vi "QuantumX_EnableBlinking.vi"(8 "Error in":errorcluster, 9 "BlinkColor":i32(ring)=2 items=["Green"=1, "Orange"=2, "Red"=3], 10 "Signal":refnum<k24>, 11 "DevicesAndSignals":T1) -> (0 "Error out":errorcluster, 3 "DevicesAndSignals":T1)   [LabVIEW 2016]
doc: "Enables blinking at the connector to which the given signal belongs.\n\nSignal: Signal, whose connector should start blinking in the given color.\nBlinkColor: Blinking color of the LED."
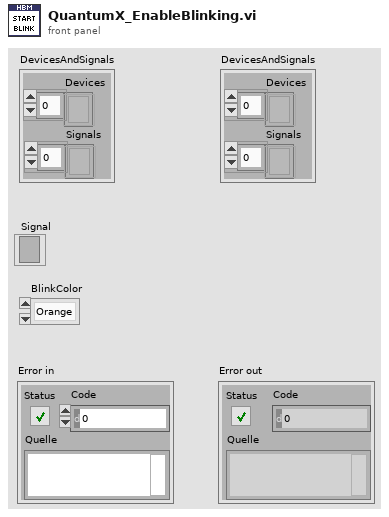
[diagram p1: front panel]
types:
  T1 = cluster{"Devices":refnum<k24>[], "Signals":refnum<k24>[]}
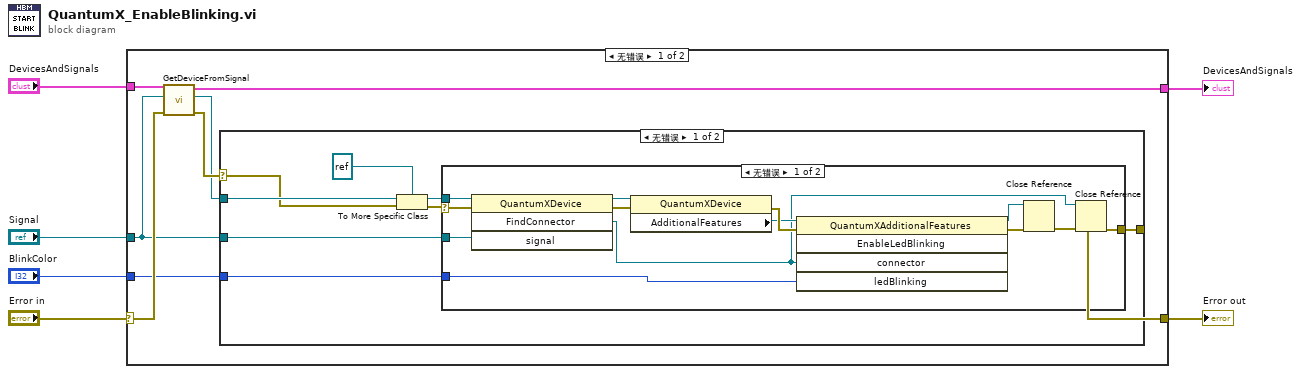
[diagram p0: block diagram]
diagram:
  n1 = case shown="无错误" "Error in" {
    selector: "Error in" -> [w13 w39]
    tunnel: "Signal" -> [w10 _]
    tunnel: "DevicesAndSignals" -> [w14 w38]
    tunnel: "BlinkColor" -> [w9 _]
    tunnel: [w8 w39] -> w2
    tunnel: [w7 w38] -> w1
    frame No Error {
      n2 = call "GetDeviceFromSignal.vi"("Error in"=w13, "Signal"=w10, "DevicesAndSignals"=w14) -> ("Error out"=w12:errorcluster, "Device"=w11:refnum<k24>, "DevicesAndSignals"=w7:T1)  [unwired: 6 in]
      n3 = case shown="无错误" w12 {
        selector: w12 -> [w16 w37]
        tunnel: w11 -> [w21 _]
        tunnel: w10 -> [w19 _]
        tunnel: w9 -> [w18 _]
        tunnel: [w17 w37] -> w8
        frame No Error {
          n4 = To More Specific Class(target class=refnum<k24> refnum (".NET (Referenz)"), reference=w21, error in=w16) -> (specific class reference=w22:refnum<k24>, error out=w20:errorcluster)
          n5 = case shown="无错误" w20 {
            selector: w20 -> [w32 w36]
            tunnel: w22 -> [w33 _]
            tunnel: w19 -> [w31 _]
            tunnel: w18 -> [w28 _]
            tunnel: [w23 w36] -> w17
            frame No Error {
              n6 = invoke on="Methodenknoten" class="QuantumXDevice" method="FindConnector"(reference=w33, error in=w32, "signal"=w31) -> (reference out=w30:refnum<k24>, error out=w29:errorcluster, "FindConnector"=w24:refnum<k24>)  [unwired: 1 in, 1 out]
              n7 = property on="Eigenschaftsknoten" class="QuantumXDevice"(reference=w30, error in=w29) -> (error out=w35:errorcluster, "AdditionalFeatures"=w34:refnum<k24>)  [unwired: 1 out]
              n8 = invoke on="Methodenknoten" class="QuantumXAdditionalFeatures" method="EnableLedBlinking"(reference=w34, error in=w35, "connector"=w24, "ledBlinking"=w28) -> (reference out=w26:refnum<k24>, error out=w27:errorcluster)  [unwired: 1 in, 3 out]
              n9 = Close Reference(reference=w26, error in (no error)=w27) -> (error out=w25:errorcluster)
              n10 = Close Reference(reference=w24, error in (no error)=w25) -> (error out=w23:errorcluster)
            }
            frame Error {
            }
          }
        }
        frame Error {
        }
      }
    }
    frame Error {
    }
  }
  "Error out" <- w2
  "DevicesAndSignals" <- w1
